vi "CRYMultiLine Get Rect.vi"(9 "Width":i32, 10 "Text In":string, 11 "[user-specified font]":T1={"Font Name:"="", "Size"=12, "Strikeout?"=FALSE, "Italic?"=FALSE, "Underline?"=FALSE, "Outline?"=FALSE, "Shadow?"=FALSE, "Bold?"=FALSE}) -> (1 "Height":i32, 2 "Text Out":string, 3 "No. Lines":u16)   [LabVIEW 2013]
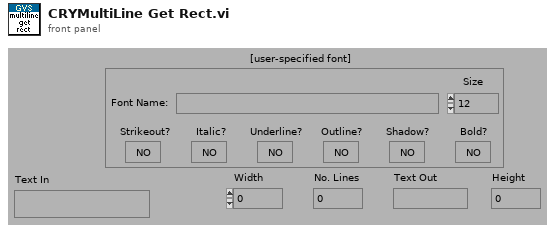
[diagram p1: front panel]
types:
  T1 = cluster{"Font Name:":string, "Size":i16, "Strikeout?":bool, "Italic?":bool, "Underline?":bool, "Outline?":bool, "Shadow?":bool, "Bold?":bool}
  T2 = enum16{"None", "Stacked", "Clockwise", "Counterclockwise"}
  T3 = cluster{"horizontal":enum16{"left", "center", "right"}, "vertical":enum16{"top", "center", "bottom"}}
  T4 = enum16{"User-specified Font", "Application Font", "System Font", "Dialog Font"}
  T5 = cluster{"left":i16, "top":i16, "right":i16, "bottom":i16}
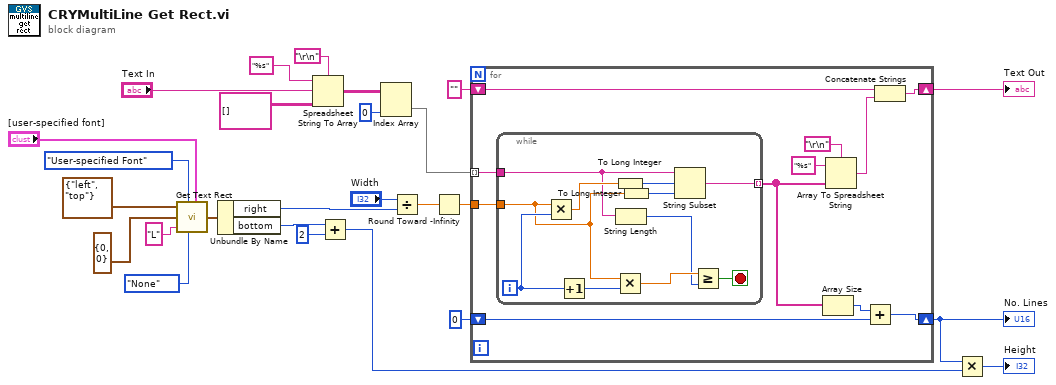
[diagram p0: block diagram]
diagram:
  n1 = call <vilib>:"Get Text Rect.vi"("alignment(left, top)"=T3 {"horizontal"=enum."left", "vertical"=enum."top"}, "desired font(Application)"=T4."User-specified Font", "origin(0,0)"=cluster{"x":i16, "y":i16} {"x"=0, "y"=0} ("origin"), "text"="L", "text orientation"=T2."None", "[user-specified font]"="[user-specified font]") -> ("rect"=w8:T5)  [unwired: 3 in]
  n2 = Unbundle By Name(w8) -> ("right"=w20:i16, "bottom"=w3:i16)
  n3 = Spreadsheet String To Array(delimiter (Tab)="\r\n", format string="%s", spreadsheet string="Text In", array type (2D Dbl)=string[][] []) -> (array=w13:string[][])
  n4 = Add(x=w3, y=i16 2) -> (x+y=w6:i16)
  n5 = Index Array(array=w13, index (col)=0 ("disabled index (col)")) -> (element=w12:string[])  [unwired: 1 in]
  n6 = Divide(x="Width", y=w20) -> (x/y=w19:dbl)
  n7 = Round Toward -Infinity(1:w19) -> (0:w18:dbl)
  n8 = for {
    tunnel: w18 -> [w37]
    tunnel: w12 -> [w36] mode=indexing
    shift-right: [w31] -> w7
    shift-left: 0 -> [w30]
    shift-right: [w28] -> w10
    shift-left: "" -> [w27]
    n9 = while {
      tunnel: w37 -> [w44]
      tunnel: [w40] -> w33 mode=indexing
      tunnel: w36 -> [w47]
      i -> [w46]
      stop <- w43 stop-if-true
      n10 = Multiply(x=w44, y=w46) -> (x*y=w48:dbl)
      n11 = Increment(x=w46) -> (x+1=w45:i32)
      n12 = To Long Integer(number=w48) -> (32bit integer=w39:i32)
      n13 = Multiply(x=w44, y=w45) -> (x*y=w42:dbl)
      n14 = String Length(string=w47) -> (length=w41:i32)
      n15 = To Long Integer(number=w44) -> (32bit integer=w38:i32)
      n16 = String Subset(string=w47, offset (0)=w39, length (rest)=w38) -> (substring=w40:string)
      n17 = Greater Or Equal?(x=w42, y=w41) -> (x >= y?=w43:bool)
    }
    n18 = Array Size(array=w33) -> (size(s)=w32:i32)
    n19 = Array To Spreadsheet String(delimiter (Tab)="\r\n", array=w33, 3:"%s" ("format string")) -> (spreadsheet string=w29:string)
    n20 = Add(x=w32, y=w30) -> (x+y=w31:i32)
    n21 = Concatenate Strings(w27, w29) -> (w28:string)
  }
  "No. Lines" <- w7
  "Text Out" <- w10
  n22 = Multiply(x=w7, y=w6) -> (x*y=→"Height":i32)
